vi "Compute Checksum.vi"(1 "Divisor":i32=8, 2 "Array":u16[](array[numeric])) -> (0 "Checksum":u8)   [LabVIEW 2019]
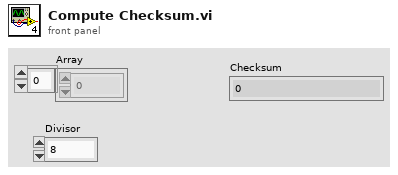
[diagram p1: front panel]
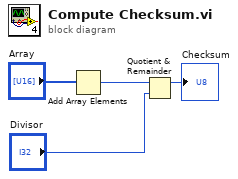
[diagram p0: block diagram]
diagram:
  n1 = Add Array Elements(numeric array="Array") -> (sum=w1:u16)
  n2 = Quotient & Remainder(x=w1, y="Divisor") -> (x-y*floor(x/y)=→"Checksum":i32)  [unwired: 1 out]
